vi "Add VIs to lvlib.vi"(6 "VIs to add":path[](array[path]), 8 "error in":errorcluster, 11 "lvlib Path":path) -> (0 "error out":errorcluster)   [LabVIEW 2026, in "NIVS_CDEW_MetaDataObj.lvclass"]
uses:
  NIVS_CDEW_MetaDataObj.lvclass
  NIVS_CDEW_MetaDataObj.lvclass/NIVS_CDEW_MetaDataObj.ctl
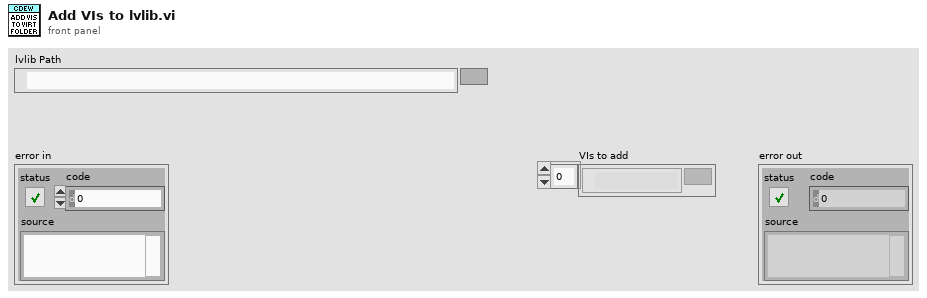
[diagram p1: front panel]
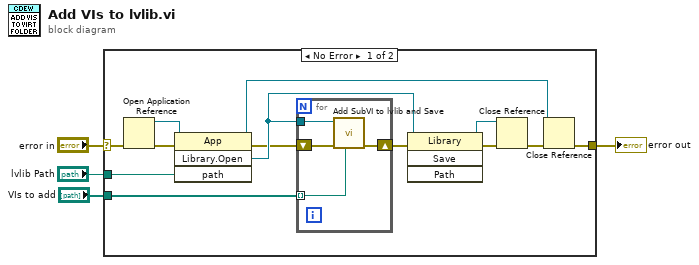
[diagram p0: block diagram]
diagram:
  n1 = case shown="No Error" "error in" {
    selector: "error in" -> [w13 w22]
    tunnel: "lvlib Path" -> [w8 _]
    tunnel: [w14 w22] -> w3
    tunnel: "VIs to add" -> [w7 _]
    frame No Error {
      n2 = Open Application Reference(8:w13) -> (0:w16:errorcluster, 3:w17:refnum<vi>)  [unwired: 3 in]
      n3 = invoke class="App" method="Library.Open"(reference=w17, error in=w16, "path"=w8) -> (reference out=w15:refnum<vi>, error out=w5:errorcluster, "Open Library"=w6:refnum<vi>)  [unwired: 1 in, 1 out]
      n4 = for {
        tunnel: w6 -> [w21]
        shift-right: [w19] -> w12
        shift-left: w5 -> [w20]
        tunnel: w7 -> [w18] mode=indexing
        n5 = call "Add SubVI to lvlib and Save.vi"("vi path"=w18, "error in"=w20, "ProjectItem"=w21) -> ("error out"=w19:errorcluster)  [unwired: 8 in]
      }
      n6 = invoke class="Library" method="Save"(reference=w6, error in=w12) -> (reference out=w9:refnum<vi>, error out=w11:errorcluster)  [unwired: 2 in, 2 out]
      n7 = Close Reference(reference=w9, error in (no error)=w11) -> (error out=w10:errorcluster)
      n8 = Close Reference(reference=w15, error in (no error)=w10) -> (error out=w14:errorcluster)
    }
    frame Error {
    }
  }
  "error out" <- w3
